vi "Histogram Comparison.vi"(8 "error in":errorcluster, 10 "Image 2":path, 11 "Image 1":path) -> (0 "error out":errorcluster, 2 "Histogram Graphs":T1, 3 "Histogram Comparison Score":dbl)   [LabVIEW 2020, in "Histogram Comparison.lvclass"]
uses:
  Histogram Comparison.lvclass
  Image Comparison/Image Comparison.lvclass
  <vilib>/Analysis/NI_AALBase.lvlib
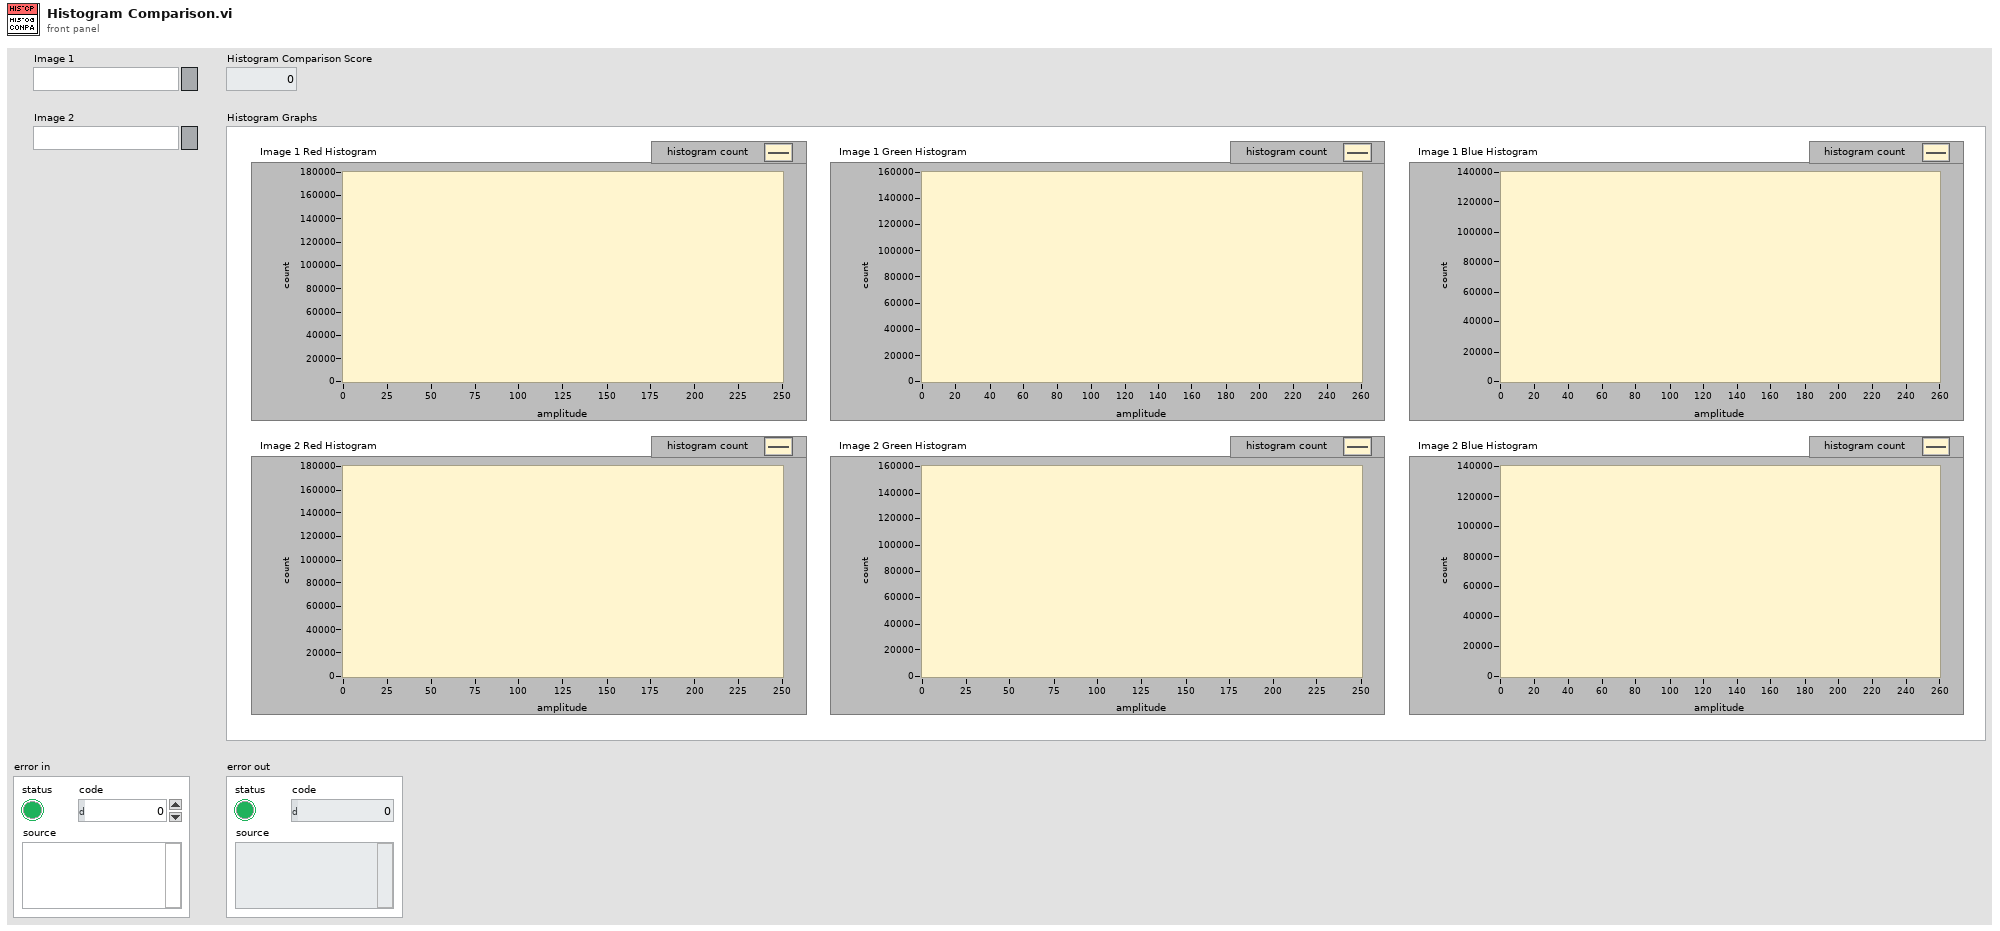
[diagram p1: front panel]
types:
  T1 = cluster{"Image 1 Red Histogram":cluster{"X Values":dbl[], "Histogram: h(x)":i32[]}, "Image 1 Green Histogram":cluster{"X Values":dbl[], "Histogram: h(x)":i32[]}, "Image 1 Blue Histogram":cluster{"X Values":dbl[], "Histogram: h(x)":i32[]}, "Image 2 Red Histogram":cluster{"X Values":dbl[], "Histogram: h(x)":i32[]}, "Image 2 Green Histogram":cluster{"X Values":dbl[], "Histogram: h(x)":i32[]}, "Image 2 Blue Histogram":cluster{"X Values":dbl[], "Histogram: h(x)":i32[]}}
  T2 = typedef "imagedata.ctl" = cluster{"image type":i32, "image depth":i32, "image":u8[], "mask":u8[], "colors":u32[], "Rectangle":cluster{"left":i16, "top":i16, "right":i16, "bottom":i16}}
  T3 = cluster{"left":i16, "top":i16, "right":i16, "bottom":i16}
  T4 = cluster{"left":u64, "top":u64, "right":u64, "bottom":u64}
  T5 = cluster{"X Values":dbl[], "Histogram: h(x)":i32[]}
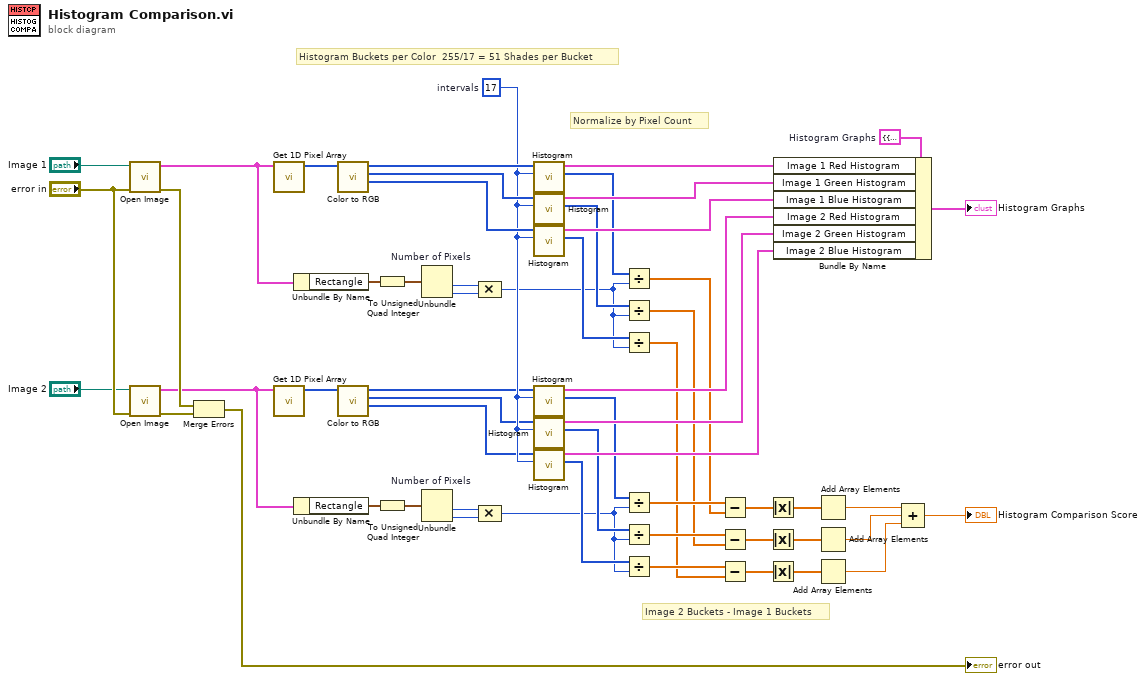
[diagram p0: block diagram]
diagram:
  w49 = T1 {"Image 1 Red Histogram"={"X Values"=[], "Histogram: h(x)"=[]}, "Image 1 Green Histogram"={"X Values"=[], "Histogram: h(x)"=[]}, "Image 1 Blue Histogram"={"X Values"=[], "Histogram: h(x)"=[]}, "Image 2 Red Histogram"={"X Values"=[], "Histogram: h(x)"=[]}, "Image 2 Green Histogram"={"X Values"=[], "Histogram: h(x)"=[]}, "Image 2 Blue Histogram"={"X Values"=[], "Histogram: h(x)"=[]}}  # Histogram Graphs
  w45 = 17  # intervals
  # "Image 2 Buckets - Image 1 Buckets"
  # "Normalize by Pixel Count"
  # "Histogram Buckets per Color  255/17 = 51 Shades per Bucket"
  n1 = call "Open Image.vi"("error in (no error)"="error in", "Image"="Image 1") -> ("error out"=w55:errorcluster, "image data"=w38:T2)  [unwired: 8 in]
  n2 = call "Open Image.vi"("error in (no error)"="error in", "Image"="Image 2") -> ("error out"=w54:errorcluster, "image data"=w31:T2)  [unwired: 8 in]
  n3 = Merge Errors(w55, w54) -> (→"error out":errorcluster)
  n4 = call "Get 1D Pixel Array.vi"("image data"=w38) -> ("1D Pixel Array"=w52:u32[])  [unwired: 10 in]
  n5 = call "Get 1D Pixel Array.vi"("image data"=w31) -> ("1D Pixel Array"=w6:u32[])  [unwired: 10 in]
  n6 = Unbundle By Name(w38) -> ("Rectangle"=w37:T3)
  n7 = Unbundle By Name(w31) -> ("Rectangle"=w32:T3)
  n8 = call "Color to RGB.vi"("1D Pixel Array"=w52) -> ("Blue[]"=w46:u8[], "Green[]"=w48:u8[], "Red[]"=w51:u8[])  [unwired: 8 in]
  n9 = call "Color to RGB.vi"("1D Pixel Array"=w6) -> ("Blue[]"=w3:u8[], "Green[]"=w4:u8[], "Red[]"=w5:u8[])  [unwired: 8 in]
  n10 = To Unsigned Quad Integer(1:w37) -> (0:w2:T4)
  n11 = To Unsigned Quad Integer(1:w32) -> (0:w1:T4)
  n12 = Unbundle "Number of Pixels"(w2) -> ("right"=w36:u64, "bottom"=w35:u64)  [unwired: 2 out]
  n13 = Unbundle "Number of Pixels"(w1) -> ("right"=w33:u64, "bottom"=w34:u64)  [unwired: 2 out]
  n14 = Compound Arithmetic op=MULTIPLY(w36, w35) -> (w27:u64)
  n15 = Compound Arithmetic op=MULTIPLY(w33, w34) -> (w23:u64)
  n16 = call <vilib>:"Histogram.vi"("intervals"=w45, "X"=w51) -> ("Histogram: h(x)"=w30:i32[], "Histogram Graph"=w50:T5)  [unwired: 6 in, 2 out]
  n17 = call <vilib>:"Histogram.vi"("intervals"=w45, "X"=w48) -> ("Histogram: h(x)"=w29:i32[], "Histogram Graph"=w47:T5)  [unwired: 6 in, 2 out]
  n18 = call <vilib>:"Histogram.vi"("intervals"=w45, "X"=w46) -> ("Histogram: h(x)"=w28:i32[], "Histogram Graph"=w44:T5)  [unwired: 6 in, 2 out]
  n19 = call <vilib>:"Histogram.vi"("intervals"=w45, "X"=w5) -> ("Histogram: h(x)"=w26:i32[], "Histogram Graph"=w43:T5)  [unwired: 6 in, 2 out]
  n20 = call <vilib>:"Histogram.vi"("intervals"=w45, "X"=w4) -> ("Histogram: h(x)"=w25:i32[], "Histogram Graph"=w42:T5)  [unwired: 6 in, 2 out]
  n21 = call <vilib>:"Histogram.vi"("intervals"=w45, "X"=w3) -> ("Histogram: h(x)"=w24:i32[], "Histogram Graph"=w41:T5)  [unwired: 6 in, 2 out]
  n22 = Divide(x=w30, y=w27) -> (x/y=w21:dbl[])
  n23 = Divide(x=w29, y=w27) -> (x/y=w19:dbl[])
  n24 = Divide(x=w28, y=w27) -> (x/y=w17:dbl[])
  n25 = Divide(x=w26, y=w23) -> (x/y=w22:dbl[])
  n26 = Divide(x=w25, y=w23) -> (x/y=w20:dbl[])
  n27 = Divide(x=w24, y=w23) -> (x/y=w18:dbl[])
  n28 = Subtract(x=w22, y=w21) -> (x-y=w16:dbl[])
  n29 = Subtract(x=w20, y=w19) -> (x-y=w15:dbl[])
  n30 = Subtract(x=w18, y=w17) -> (x-y=w14:dbl[])
  n31 = Absolute Value(x=w16) -> (abs(x)=w13:dbl[])
  n32 = Absolute Value(x=w15) -> (abs(x)=w12:dbl[])
  n33 = Absolute Value(x=w14) -> (abs(x)=w11:dbl[])
  n34 = Bundle By Name(cluster=w49, "Image 1 Red Histogram"=w50, "Image 1 Green Histogram"=w47, "Image 1 Blue Histogram"=w44, "Image 2 Red Histogram"=w43, "Image 2 Green Histogram"=w42, "Image 2 Blue Histogram"=w41) -> (→"Histogram Graphs":T1)
  n35 = Add Array Elements(numeric array=w13) -> (sum=w10:dbl)
  n36 = Add Array Elements(numeric array=w12) -> (sum=w9:dbl)
  n37 = Add Array Elements(numeric array=w11) -> (sum=w8:dbl)
  n38 = Compound Arithmetic op=ADD(w10, w9, w8) -> (→"Histogram Comparison Score":dbl)
